vi "Creator Queue Alias.vi"(11 "Base Queue in":refnum<class "Base Queue.lvclass">) -> (2 "Creator Queue Alias":string, 3 "Base Queue out":refnum<class "Base Queue.lvclass">)   [LabVIEW 2021, in "jettl.lvlib" / "Base Queue.lvlib" / "Base Queue.lvclass"]
uses:
  Base Queue.lvclass
  C:/git/jettl/src/jettl/jettl/jettl.lvclass
  Base Queue.lvclass/Base Queue.ctl
  Queue Mailbox/Queue Mailbox.lvlib
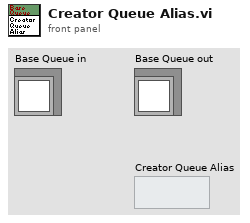
[diagram p1: front panel]
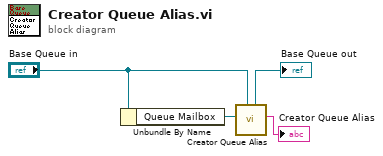
[diagram p0: block diagram]
diagram:
  n1 = Unbundle By Name("Base Queue in") -> ("Queue Mailbox"=w3:refnum<data-value>)
  n2 = call "Creator Queue Alias.vi"("jettl in"="Base Queue in", "Queue Mailbox"=w3) -> ("Creator Queue Alias"=→"Creator Queue Alias":string, "jettl out"=→"Base Queue out":refnum<class "Base Queue.lvclass">)  [unwired: 8 in]
